vi "UDP receiver_queue_2.vi"(11 "dup Message Queue":refnum<queue>) -> ()   [LabVIEW 2017]
uses:
  UI Error Handlers/support/Logging/Control 2.ctl
  UI Error Handlers/support/Message Queue/Message Cluster.ctl
  Globals/Global - Configuration Options.vi
  UI Error Handlers/support/Logging/Logging.lvlib
  UI Error Handlers/support/Message Queue/Message Queue.lvlib
panel:
  out "x-y":u32
  out "error out 2":errorcluster
  in  "?":T1
  out "error out":errorcluster
  in  "stop":bool
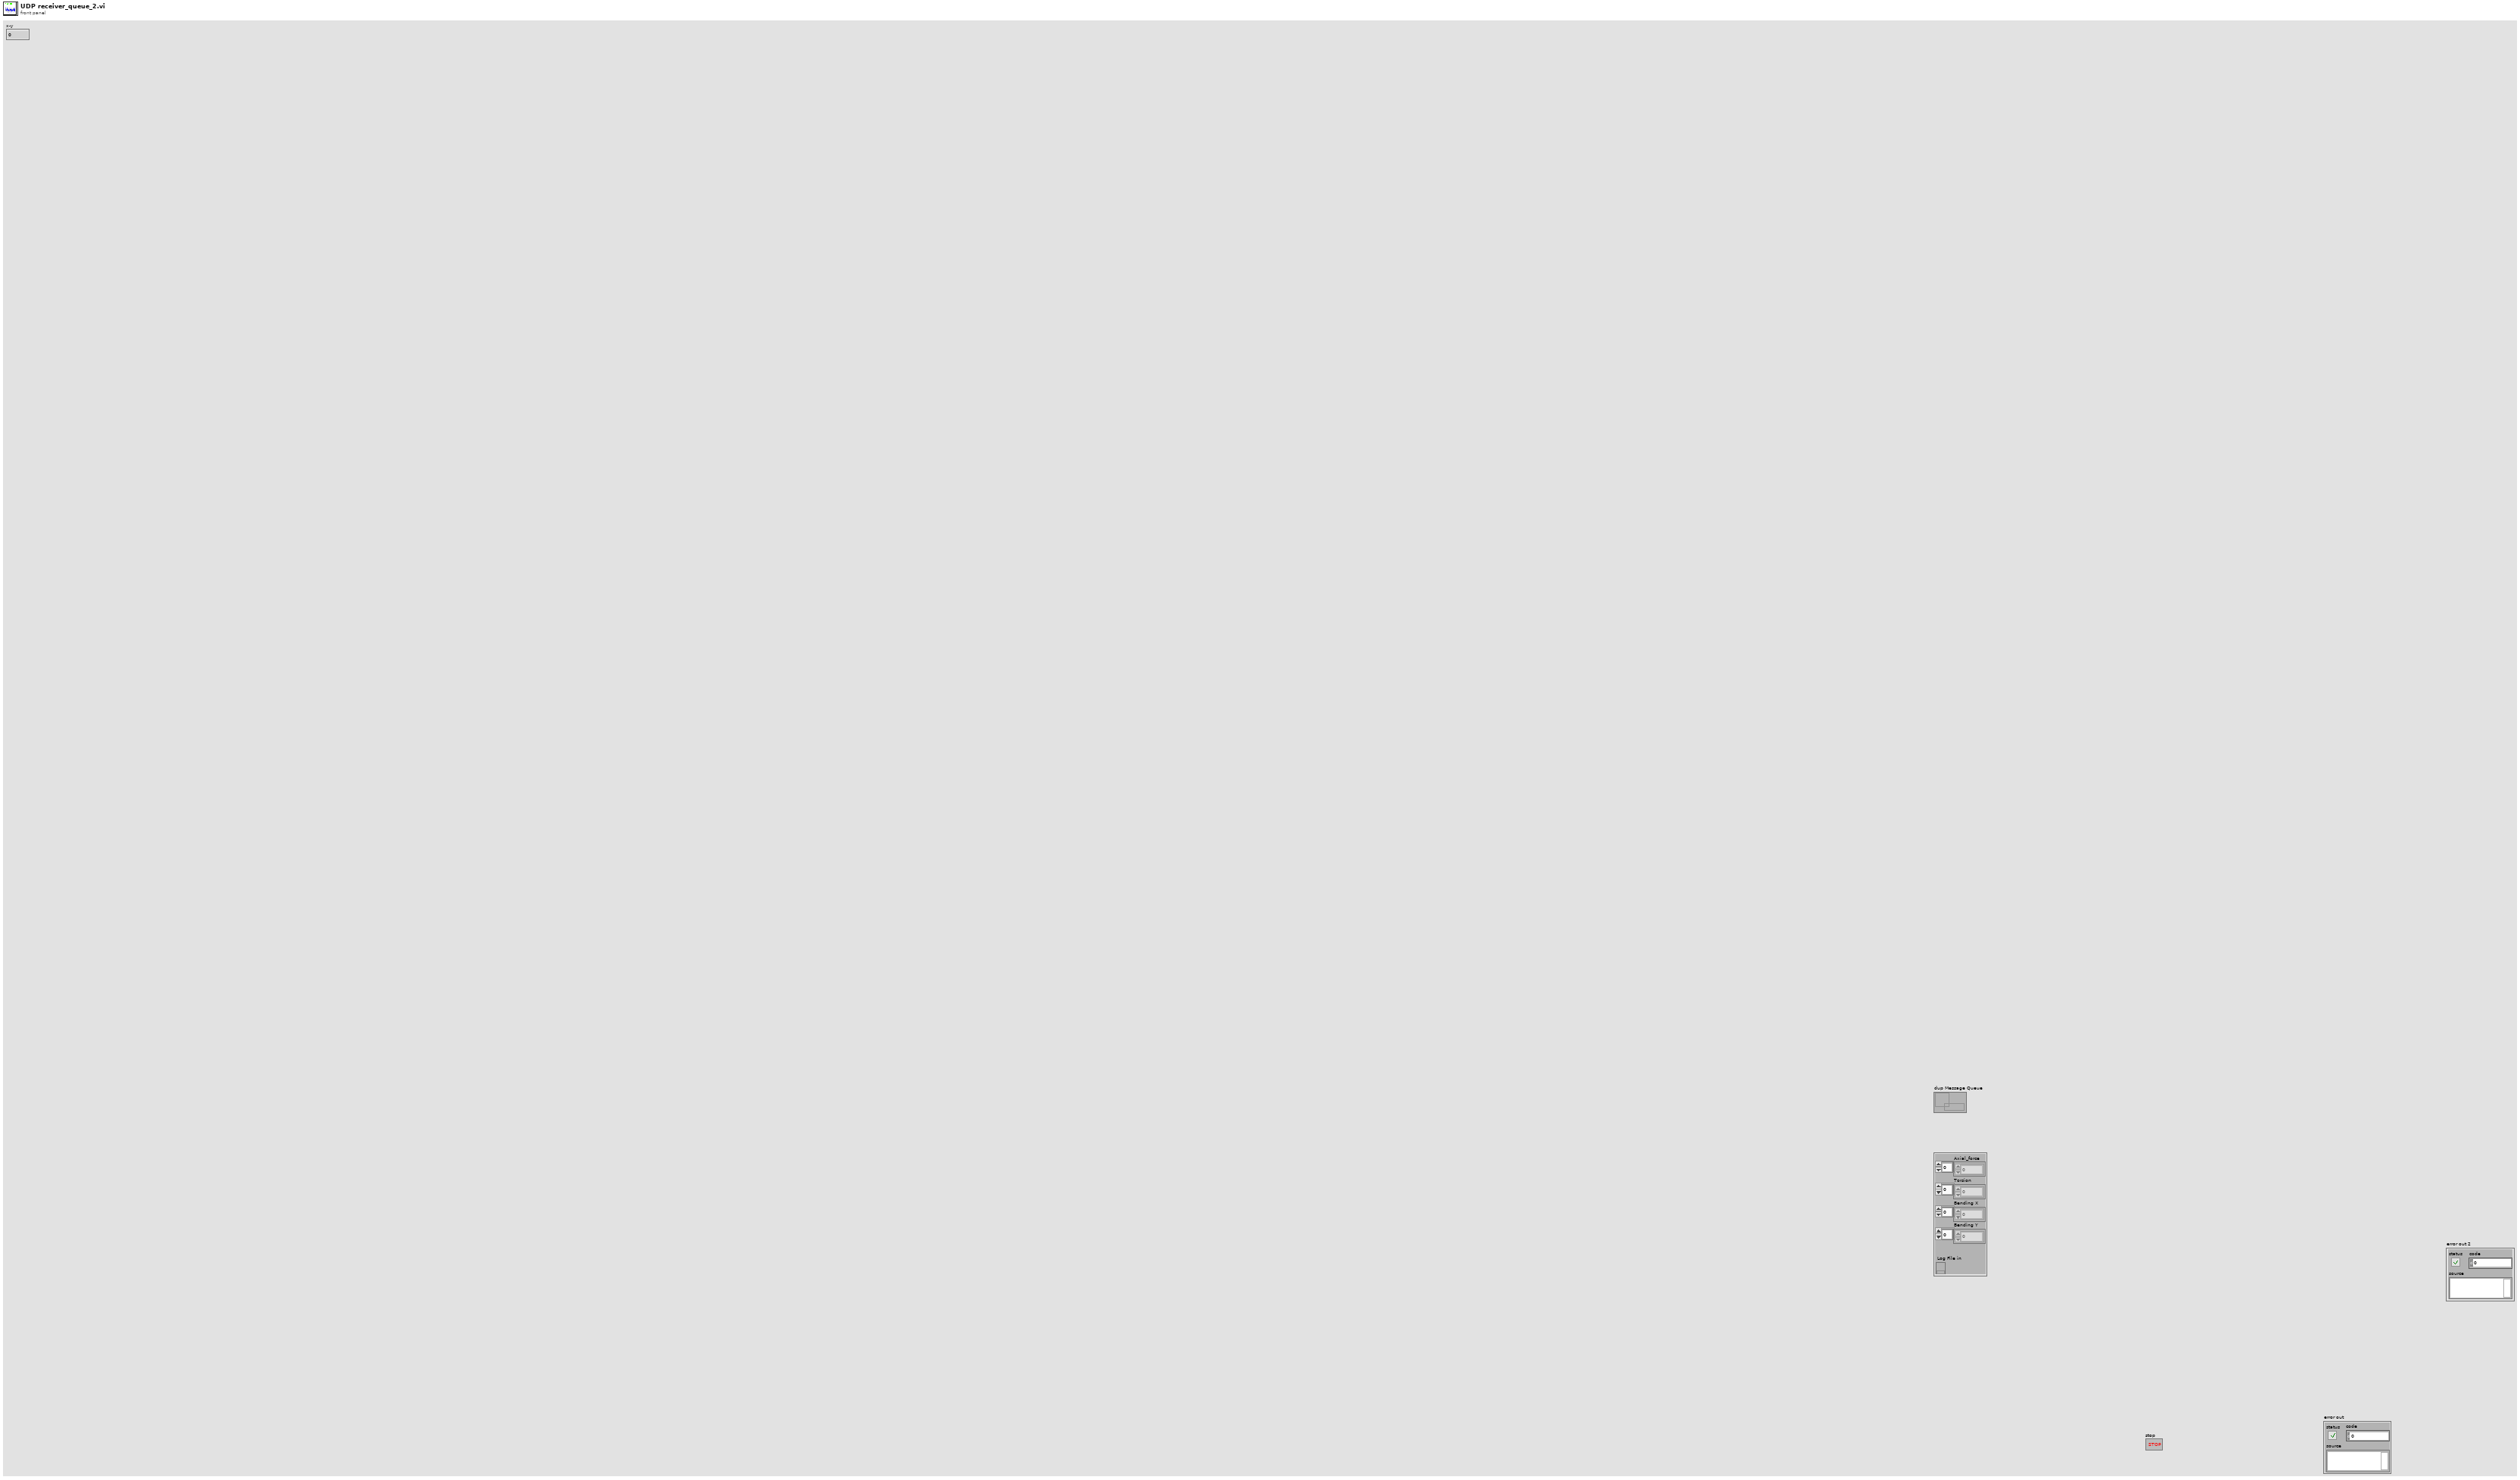
[diagram p1: front panel]
types:
  T1 = typedef "Control 2.ctl" = cluster{"Axial_force":i16[], "Torsion":i16[], "Bending X":i16[], "Bending Y":i16[], "Log File in":refnum<k34>}
  T2 = cluster{"Tool data":cluster{"Number of teeth":sgl}, "Cutting data":cluster{"rpm":sgl}, "Limits":cluster{"Magnitude threshold":sgl, "Tolerance":sgl}, "G1 status":cluster{"G1 trigger":bool}}
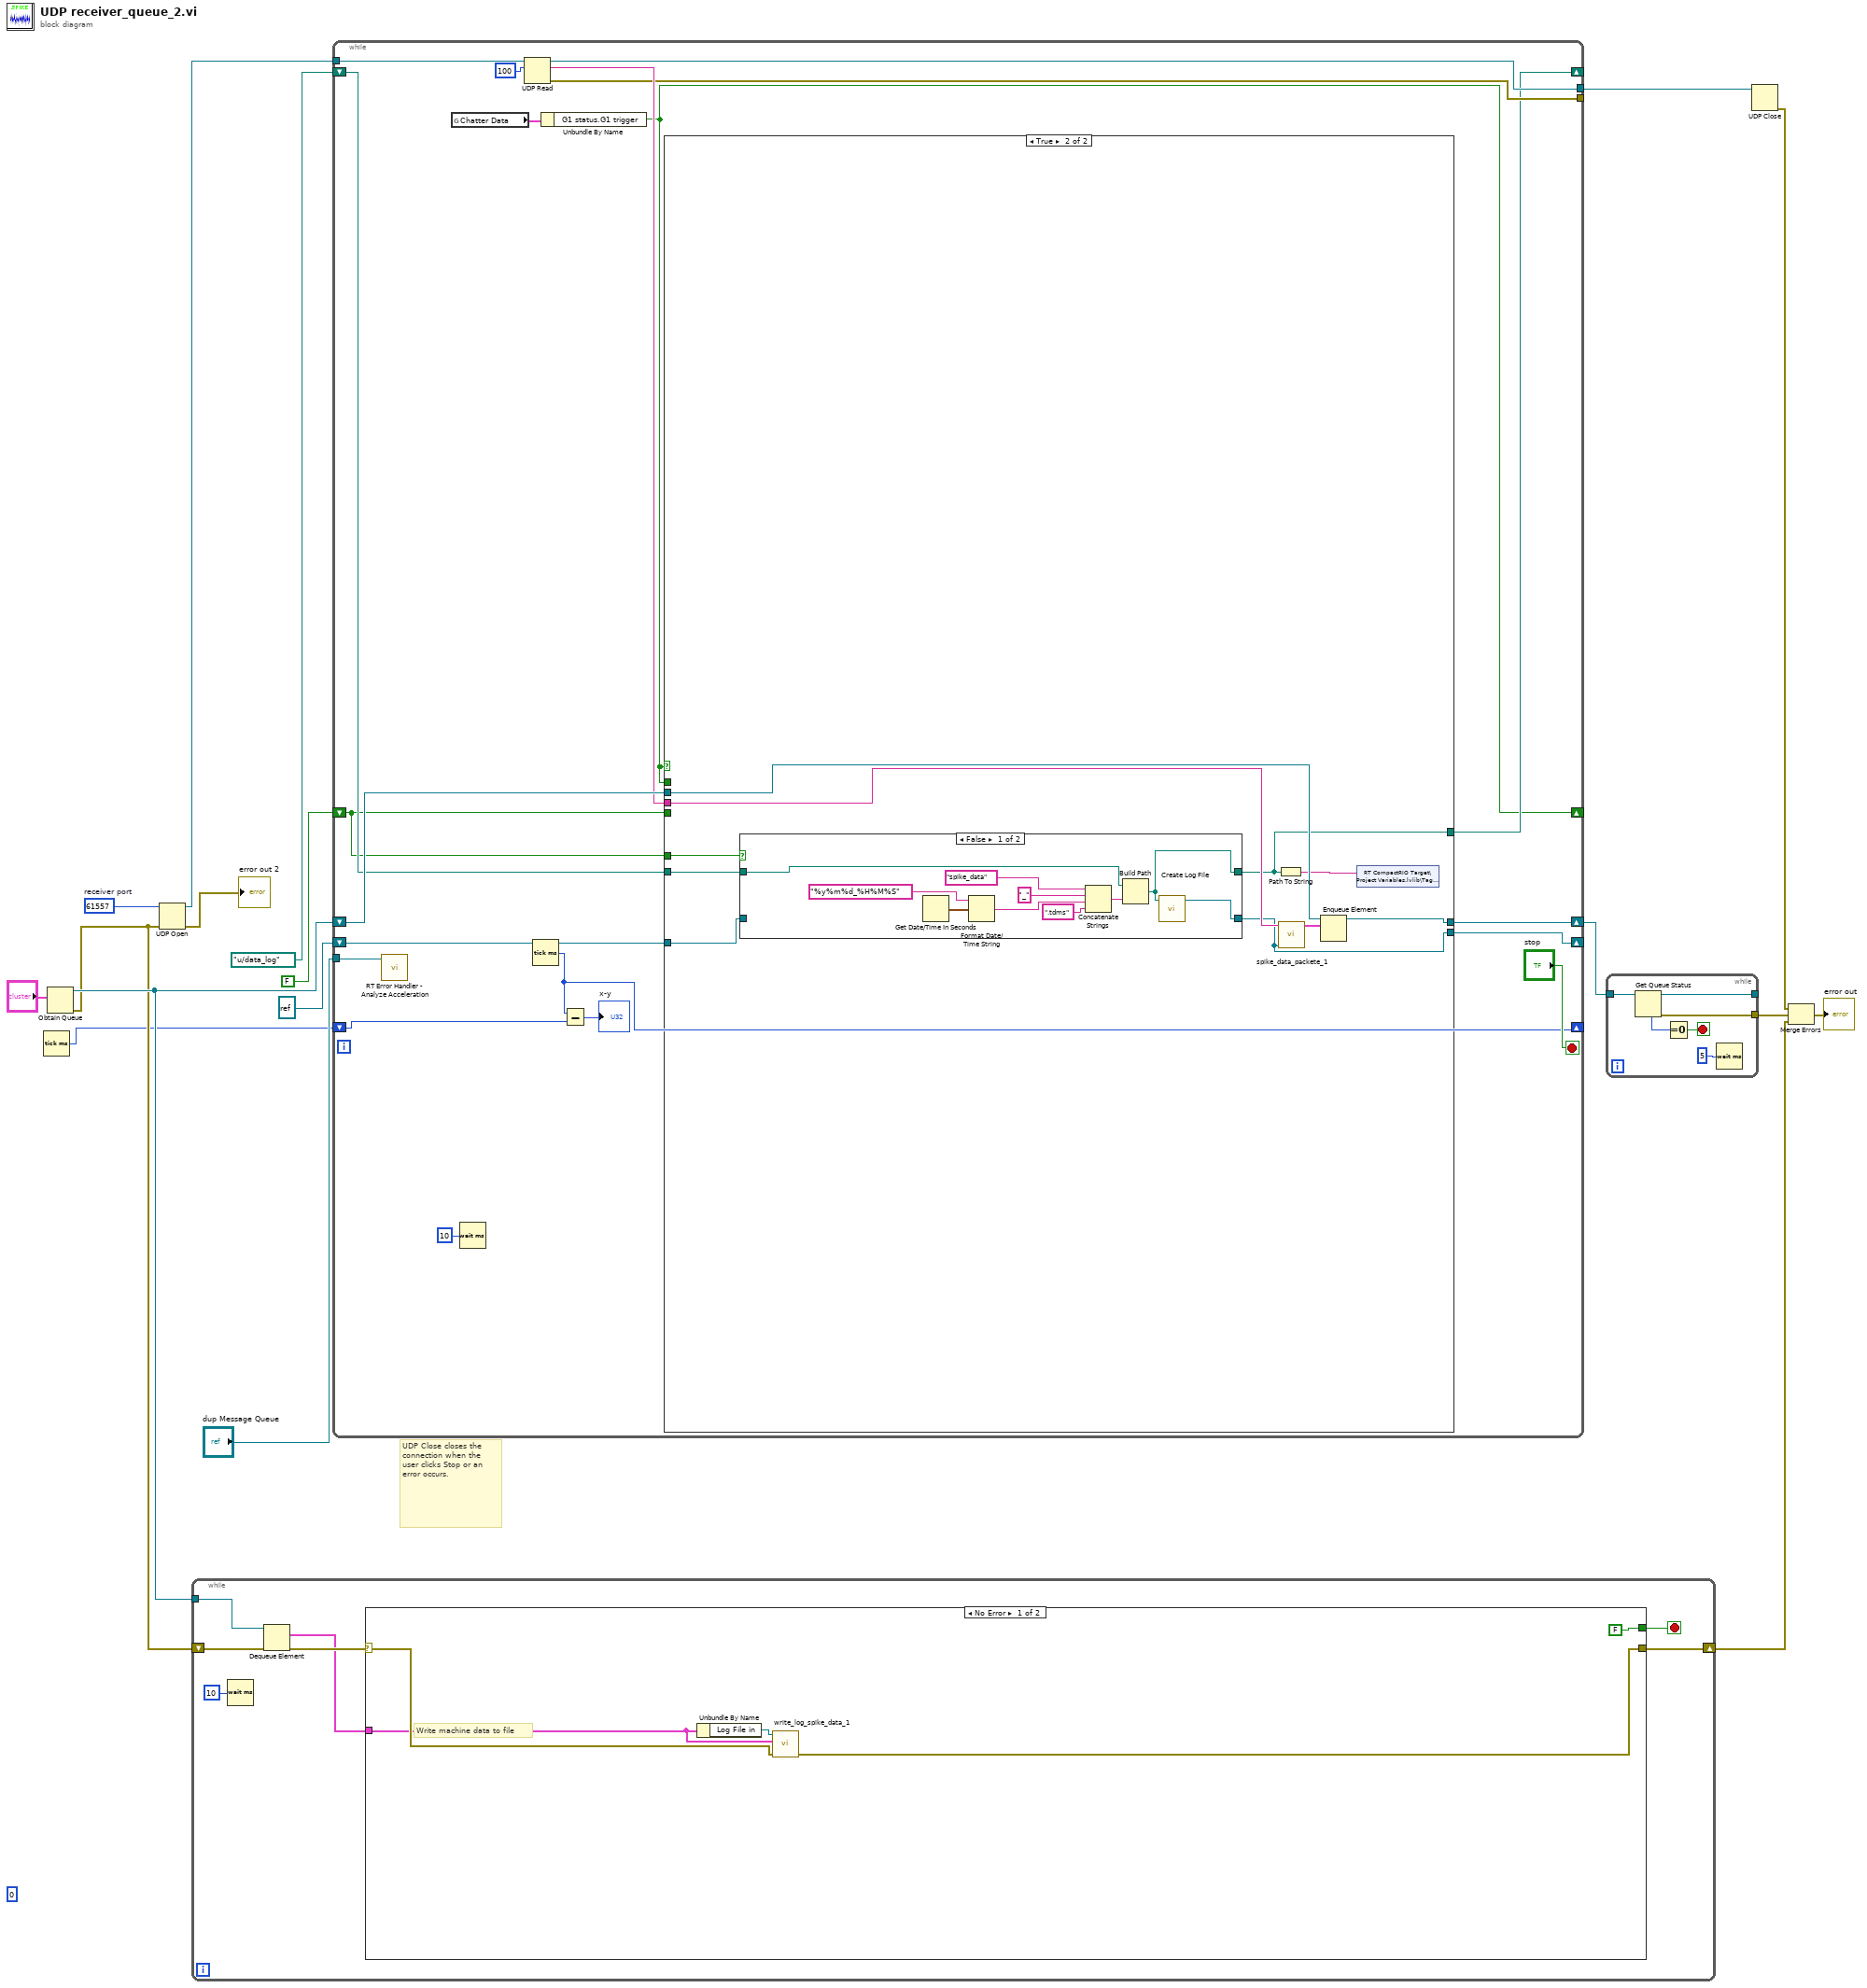
[diagram p0: block diagram]
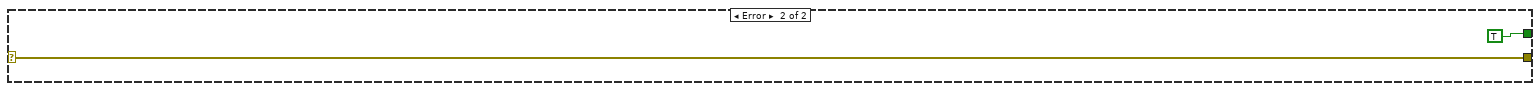
[diagram p2: hidden frame]
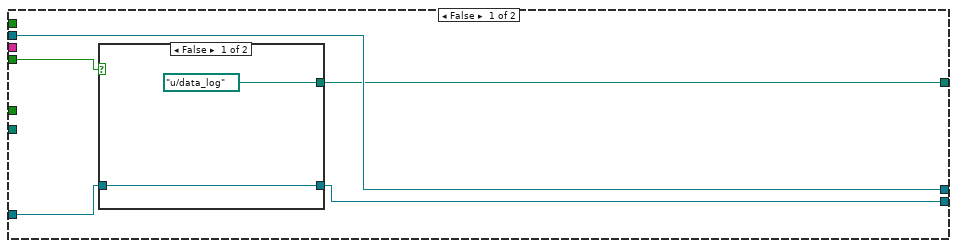
[diagram p3: hidden frame]
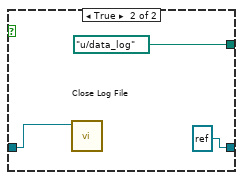
[diagram p4: hidden frame]
diagram:
  (unwired) i16 0 ("A(I16) 11")
  w17 = u16 61557  # receiver port
  # "UDP Close closes the connection when the user clicks Stop or an error occurs."
  n1 = Tick Count (ms)() -> (millisecond timer value=w1:u32)
  n2 = Obtain Queue(element data type="?") -> (queue out=w13:refnum<queue>, error out=w2:errorcluster)  [unwired: 4 in, 1 out]
  n3 = UDP Open(8:w2, 11:w17) -> (port=w16:refnum<k16>, 0:→"error out 2":errorcluster)  [unwired: 3 in, 1 out]
  n4 = while {
    tunnel: w13 -> [w24]
    shift-right: [w20] -> w12
    shift-left: w2 -> [w23]
    stop <- w21 stop-if-true
    n5 = Wait (ms)(milliseconds to wait=u32 10) -> ()  [unwired: 1 out]
    n6 = Dequeue Element(queue=w24, error in (no error)=w23) -> (element=w19:T1, error out=w22:errorcluster)  [unwired: 1 in, 2 out]
    n7 = case shown="No Error" w22 {
      selector: w22 -> [w27 w30]
      tunnel: [FALSE TRUE] -> w21
      tunnel: [w25 w30] -> w20
      tunnel: w19 -> [w26 _]
      frame No Error {
        # "Write machine data to file"
        n8 = Unbundle By Name(w26) -> ("Log File in"=w28:refnum<k34>)
        n9 = call "write_log_spike_data_1.vi"("error in (no error)"=w27, "Cluster 2"=w26, "Log File in"=w28) -> ("error out"=w25:errorcluster)  [unwired: 7 in, 1 out]
      }
      frame Error {
      }
    }
  }
  n10 = while {
    tunnel: w16 -> [w50]
    shift-right: [w43] -> w15
    shift-left: w13 -> [w51]
    tunnel: [w47] -> w10
    shift-right: [w41] -> _
    shift-left: refnum<k34> refnum ("Log File out") -> [w39]
    shift-right: [w42] -> _
    shift-left: path "u:/data_log" ("AVI Path") -> [w45]
    shift-right: [w36] -> _
    shift-left: FALSE -> [w40]
    tunnel: [w44] -> _
    tunnel: "dup Message Queue" -> [w38]
    shift-right: [w33] -> _
    shift-left: w1 -> [w34]
    stop <- "stop" stop-if-true
    n11 = call "RT Error Handler - Analyze Acceleration.vi"("Message Queue"=w38) -> ()  [unwired: 10 in, 1 out]
    n12 = global read "Global - Configuration Options.vi" "Chatter Data"() -> (w37:T2)
    n13 = Wait (ms)(milliseconds to wait=u32 10) -> ()  [unwired: 1 out]
    n14 = UDP Read(connection ID=w50, max size (548)=100 ("timeout ms (25000)")) -> (data out=w48:string, error out=w44:errorcluster, 3:w47:refnum<k16>)  [unwired: 2 in, 2 out]
    n15 = Tick Count (ms)() -> (millisecond timer value=w33:u32)
    n16 = Unbundle By Name(w37) -> ("G1 status.G1 trigger"=w36:bool)
    n17 = Subtract(x=w33, y=w34) -> (x-y=→"x-y":u32)
    n18 = case shown="True" w36 {
      tunnel: w51 -> [w56 w71]
      tunnel: [w56 w70] -> w43
      tunnel: w48 -> [_ w66]
      tunnel: w36 -> [_ _]
      tunnel: w45 -> [_ w69]
      tunnel: [w53 w64] -> w42
      tunnel: [w52 w65] -> w41
      tunnel: w39 -> [w54 w68]
      tunnel: w40 -> [_ w67]
      tunnel: w40 -> [w55 _]
      frame False {
        n19 = case shown="False" w55 {
          tunnel: [path "u:/data_log" ("AVI Path") path "u:/data_log" ("AVI Path")] -> w53
          tunnel: [w57 refnum<k34> refnum ("Log File out")] -> w52
          tunnel: w54 -> [w57 w59]
          frame False {
          }
          frame True {
            n20 = call "Close Log File.vi"("tdms file"=w59) -> ()  [unwired: 10 in, 1 out]
          }
        }
      }
      frame True {
        n21 = case shown="False" w67 {
          tunnel: [w74 w83] -> w64
          tunnel: [w73 w82] -> w65
          tunnel: w69 -> [w72 w83]
          tunnel: w68 -> [_ w82]
          frame False {
            n22 = Get Date/Time In Seconds() -> (seconds since 1Jan1904=w77:timestamp)
            n23 = Format Date/Time String(time format string (%c)="%y%m%d_%H%M%S", seconds (now)=w77) -> (date/time string=w80:string)  [unwired: 1 out]
            n24 = Concatenate Strings("spike_data" ("string"), "_" ("string"), w80, ".tdms" ("string")) -> (w75:string)
            n25 = Build Path(base path=w72, name or relative path=w75) -> (appended path=w74:path)
            n26 = call "Create Log File.vi"("Acceleration Exceeded Log Folder"=w74) -> ("Log File out"=w73:refnum<k34>)  [unwired: 9 in, 1 out]
          }
          frame True {
          }
        }
        n27 = Path To String(path=w64) -> (string=w63:string)
        n28 = call "spike_data_packete_1.vi"("Log File in"=w65, "data out"=w66) -> ("output cluster"=w62:T1)  [unwired: 9 in]
        n29 = Enqueue Element(queue=w71, element=w62) -> (queue out=w70:refnum<queue>)  [unwired: 2 in, 2 out]
        n30 = shared-variable "RT CompactRIO Target\\Project Variables.lvlib\\Tag Video"(w63) -> ()  [unwired: 1 in, 1 out]
      }
    }
  }
  n31 = while {
    tunnel: [w88] -> w14
    tunnel: [w86] -> _
    tunnel: w15 -> [w84]
    stop <- w87 stop-if-true
    n32 = Get Queue Status(queue=w84) -> (queue out=w86:refnum<queue>, error out=w88:errorcluster, # elements in queue=w85:i32)  [unwired: 2 in, 5 out]
    n33 = Equal To 0?(x=w85) -> (x = 0?=w87:bool)
    n34 = Wait (ms)(milliseconds to wait=u32 5) -> ()  [unwired: 1 out]
  }
  n35 = UDP Close(connection ID=w10) -> (error out=w9:errorcluster)  [unwired: 1 in, 1 out]
  n36 = Merge Errors(w9, w14, w12) -> (→"error out":errorcluster)
